vi "Plotmatrix Property Dialog.vi"(6 "Control Ref Queue":T9, 7 "Multimatrix Representation":T10, 8 "error in (no error)":errorcluster, 11 "2D Feather.lvclass in":refnum<class "XY Plot Matrix.lvclass">) -> (0 "error out":errorcluster, 3 "2D Feather.lvclass out":refnum<class "XY Plot Matrix.lvclass">, 4 "Cancel?":bool)   [LabVIEW 2020, in "XY Plot Matrix.lvclass"]
uses:
  <vilib>/Math Plots/2D Math Plots/XY Plot Matrix/XY Plot Matrix/XY Plot Matrix.lvclass
  e:/builds/penguin/labview/branches/2020/dev/dist/vi.lib/Math Plots/2D Math Plots/2D Plot/2D Plot/2D Plot.lvclass
  <vilib>/Math Plots/2D Math Plots/2D Plot/Action String/XYPlotMatrix Ctrl Act Queue.ctl
  <vilib>/Math Plots/2D Math Plots/2D Plot/Action String/XYPlotMatrix Ctrl Act Cluster.ctl
  <vilib>/Math Plots/2D Math Plots/2D Plot/Action String/2DMathPlot State Class.ctl
  <vilib>/Math Plots/2D Math Plots/2D Plot/2D Plot/Typedef/Scale Cluster.ctl
  <vilib>/Utility/miscctls.llb/LVOffsetAndMultiplierTypeDef.ctl
  <vilib>/Math Plots/2D Math Plots/XY Plot Matrix/XY Plot Matrix/Typedef/Plotmatrix Property Array.ctl
  <vilib>/Math Plots/2D Math Plots/XY Plot Matrix/XY Plot Matrix/Typedef/Plotmatrix Property.ctl
  <vilib>/Math Plots/2D Math Plots/2D Plot/2D Plot/Typedef/Plot Property Array.ctl
  <vilib>/Math Plots/2D Math Plots/2D Plot/2D Plot/Typedef/Plot Property.ctl
  <vilib>/Math Plots/2D Math Plots/2D Plot/2D Plot/Typedef/Graph General Property.ctl
  <vilib>/Math Plots/2D Math Plots/XY Plot Matrix/XY Plot Matrix/Typedef/Mulitmatrix Representation.ctl
  <vilib>/Math Plots/2D Math Plots/XY Plot Matrix/XY Plot Matrix/Typedef/Matrix Representation.ctl
  <vilib>/Math Plots/2D Math Plots/2D Plot/2D Plot/Typedef/Range Cluster.ctl
  <vilib>/Math Plots/2D Math Plots/2D Plot/2D Plot/Typedef/Temp Graph State.ctl
  <vilib>/Math Plots/2D Math Plots/2D Plot/2D Plot/Typedef/Temp Graph Data Action.ctl
  <vilib>/Math Plots/2D Math Plots/XY Plot Matrix/XY Plot Matrix/XY Plot Matrix.lvclass/XY Plot Matrix.ctl
  <vilib>/Math Plots/2D Math Plots/2D Plot/2D Plot/2D Plot.lvclass
panel:
  in  "Graph General":T1
  in  "Format String":string[](array[string])
  in  "Plotmatrix Property":T2
  in  "Scales Array":T6[](array[typedef])
  in  "Dialog Tab":enum32{"UI", "Input & Output"}(tab)
  in  "OK":bool
  in  "Cancel":bool
  in  "Help":bool
  in  "Page Tab":T8(tab)
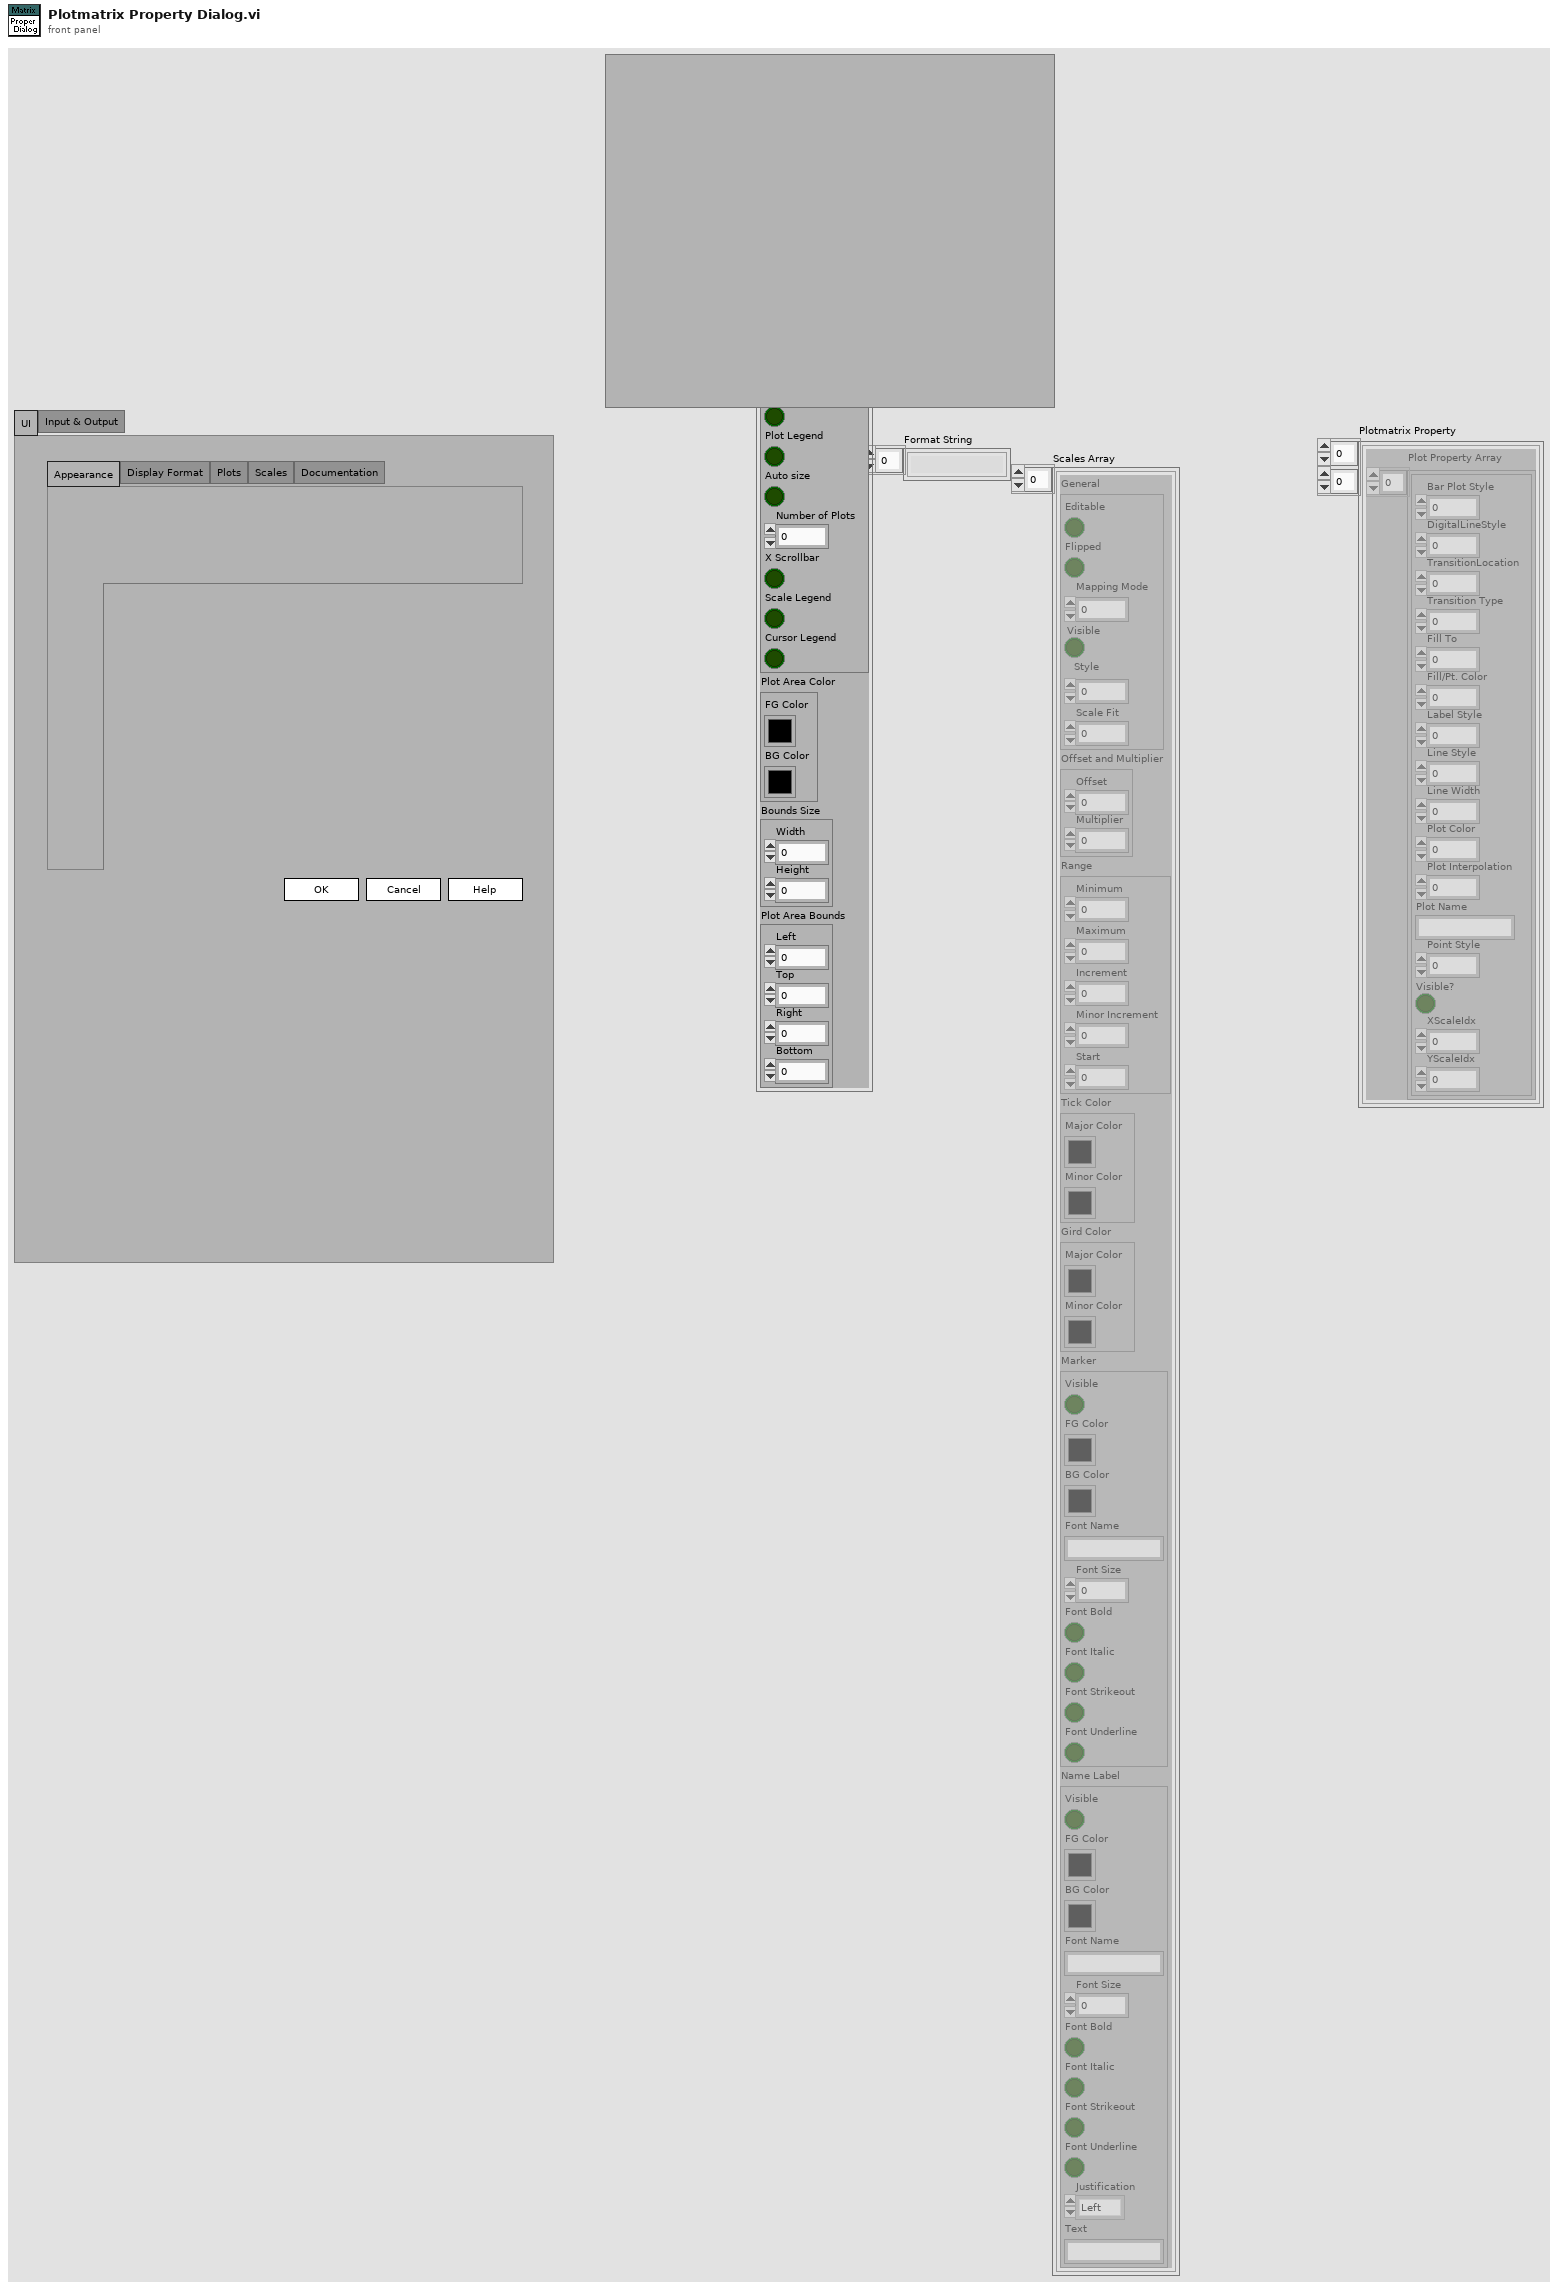
[diagram p1: front panel]
types:
  T1 = typedef "2D Plot.lvclass/Graph General Property.ctl" = cluster{"Palette Visible":cluster{"Graph Legend":bool, "Plot Legend":bool, "Auto size":bool, "Number of Plots":u32, "X Scrollbar":bool, "Scale Legend":bool, "Cursor Legend":bool}, "Plot Area Color":cluster{"FG Color":u32, "BG Color":u32}, "Bounds Size":cluster{"Width":u32, "Height":u32}, "Plot Area Bounds":cluster{"Left":i16, "Top":i16, "Right":i16, "Bottom":i16}}
  T2 = typedef "XY Plot Matrix.lvclass/Plotmatrix Property Array.ctl" = T3[][]
  T3 = typedef "XY Plot Matrix.lvclass/Plotmatrix Property.ctl" = cluster{"Plot Property Array":T4}
  T4 = typedef "2D Plot.lvclass/Plot Property Array.ctl" = T5[]
  T5 = typedef "2D Plot.lvclass/Plot Property.ctl" = cluster{"Bar Plot Style":u8, "DigitalLineStyle":u8, "TransitionLocation":u8, "Transition Type":u8, "Fill To":i16, "Fill/Pt. Color":u32, "Label Style":u8, "Line Style":u8, "Line Width":u8, "Plot Color":u32, "Plot Interpolation":u8, "Plot Name":string, "Point Style":u8, "Visible?":bool, "XScaleIdx":u32, "YScaleIdx":u32}
  T6 = typedef "2D Plot.lvclass/Scale Cluster.ctl" = cluster{"General":cluster{"Editable":bool, "Flipped":bool, "Mapping Mode":u8, "Visible":bool, "Style":u8, "Scale Fit":u8}, "Offset and Multiplier":T7, "Range":cluster{"Minimum":dbl, "Maximum":dbl, "Increment":dbl, "Minor Increment":dbl, "Start":dbl}, "Tick Color":cluster{"Major Color":u32, "Minor Color":u32}, "Gird Color":cluster{"Major Color":u32, "Minor Color":u32}, "Marker":cluster{"Visible":bool, "FG Color":u32, "BG Color":u32, "Font Name":string, "Font Size":u32, "Font Bold":bool, "Font Italic":bool, "Font Strikeout":bool, "Font Underline":bool}, "Name Label":cluster{"Visible":bool, "FG Color":u32, "BG Color":u32, "Font Name":string, "Font Size":u32, "Font Bold":bool, "Font Italic":bool, "Font Strikeout":bool, "Font Underline":bool, "Justification":enum16{"Left", "Center", "Right"}, "Text":string}}
  T7 = typedef "LVOffsetAndMultiplierTypeDef.ctl" = cluster{"Offset":dbl, "Multiplier":dbl}
  T8 = enum32{"Appearance", "Display Format", "Plots", "Scales", "Documentation"}
  T9 = typedef "XYPlotMatrix Ctrl Act Queue.ctl" = refnum<queue>
  T10 = typedef "XY Plot Matrix.lvclass/Mulitmatrix Representation.ctl" = cluster{"Matrix Representation Array":T11[][], "Max Range Array":T12[][], "Max Plot Number":i32}
  T11 = typedef "XY Plot Matrix.lvclass/Matrix Representation.ctl" = cluster{"Graph Matrix":cluster{"X":dbl[], "Y":dbl[]}[]}
  T12 = typedef "2D Plot.lvclass/Range Cluster.ctl" = cluster{"X Range":cluster{"Max X":dbl, "Min X":dbl}, "Y Range":cluster{"Max Y":dbl, "Min Y":dbl}}
  T13 = typedef "2D Plot.lvclass/Temp Graph State.ctl" = enum16{"Create", "Update Graph", "Update Property Only", "Get Plot Name", "Get Axis Name", "Destory"}
  T14 = typedef "2D Plot.lvclass/Temp Graph Data Action.ctl" = enum16{"Data Cluster", "Property Class", "Control Queue"}
  T15 = typedef "XYPlotMatrix Ctrl Act Cluster.ctl" = cluster{"Facade VI":refnum<vi>, "XControl":refnum<vi>, "Sub Panel":refnum<vi>, "Sub VI":refnum<vi>, "Export Image":refnum<vi>, "Display State Change Class":T16}
  T16 = typedef "2DMathPlot State Class.ctl" = enum16{"Update All (Undo)", "Update General", "Update Appearance", "Update Format", "Update Scale", "Update Marker", "Update Cursor", "None"}
  T17 = typedef "2D Plot.lvclass/Property Cluster.ctl" = cluster{"Graph General":T1, "Format Property":string[], "Scale Array":T18, "Cursor Property":T19, "Annotation List":T21, "Active Cursor":i32, "Active Plot":i32}
  T18 = typedef "2D Plot.lvclass/Scale Array.ctl" = T6[]
  T19 = typedef "2D Plot.lvclass/Cursor Property.ctl" = cluster{"Cursor List":T20, "Cursor List Addtional":cluster{"Cursor Selection Color":u32, "Line Style":u8, "Line Width":u8, "Visible":bool}[]}
  T20 = typedef "LVCursorListTypeDef.ctl" = cluster{"Name":string, "Color":u32, "Style":u8, "Point Style":u8, "Name Visible":bool, "Allow Drag":bool, "Cursor Mode":u32, "Plot":i32, "Index":i32, "Position":cluster{"X":dbl, "Y":dbl}, "X Scale":u32, "Y Scale":u32, "Watch Plots":i32[], "Watch All Plots":bool, "Plot Area":i32, "Label Offset":cluster{"X":dbl, "Y":dbl}}[]
  T21 = typedef "LVAnnotationListTypeDef.ctl" = cluster{"Name":string, "Color":u32, "Style":u8, "Point Style":u8, "Name Visible":bool, "Allow Drag":bool, "Annotation Mode":u32, "Plot":i32, "Index":i32, "Position":cluster{"X":dbl, "Y":dbl}, "X Scale":u32, "Y Scale":u32, "Show Arrow":bool, "Lock Name":bool, "Plot Area":i32, "Label Offset":cluster{"X":dbl, "Y":dbl}}[]
  T22 = enum8{"Enabled", "Disabled", "Disabled and Grayed Out"}
  T23 = enum32{"Bad", "Idle", "Run top level", "Running"}[]
  T24 = enum32{"Bad", "Idle", "Run top level", "Running"}
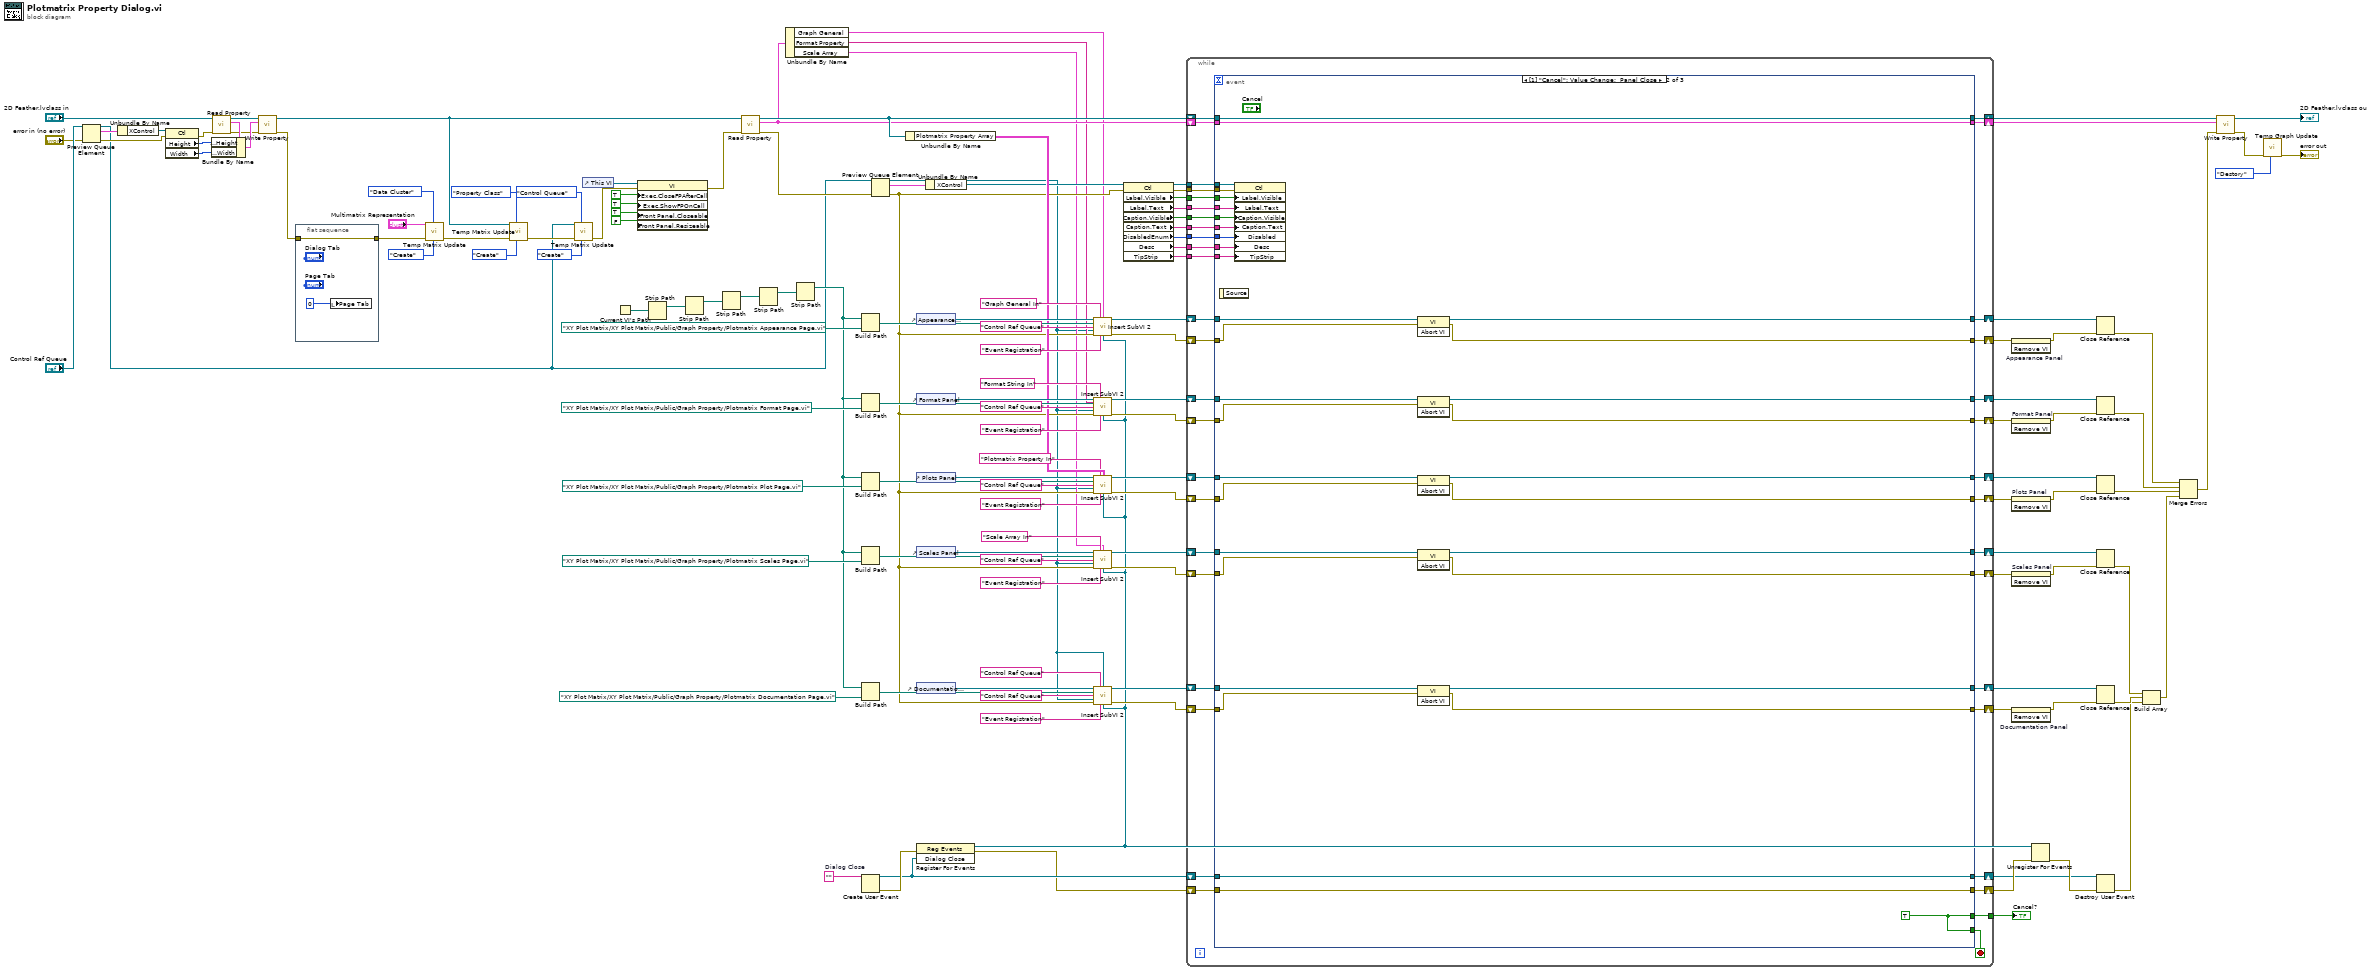
[diagram p0: block diagram]
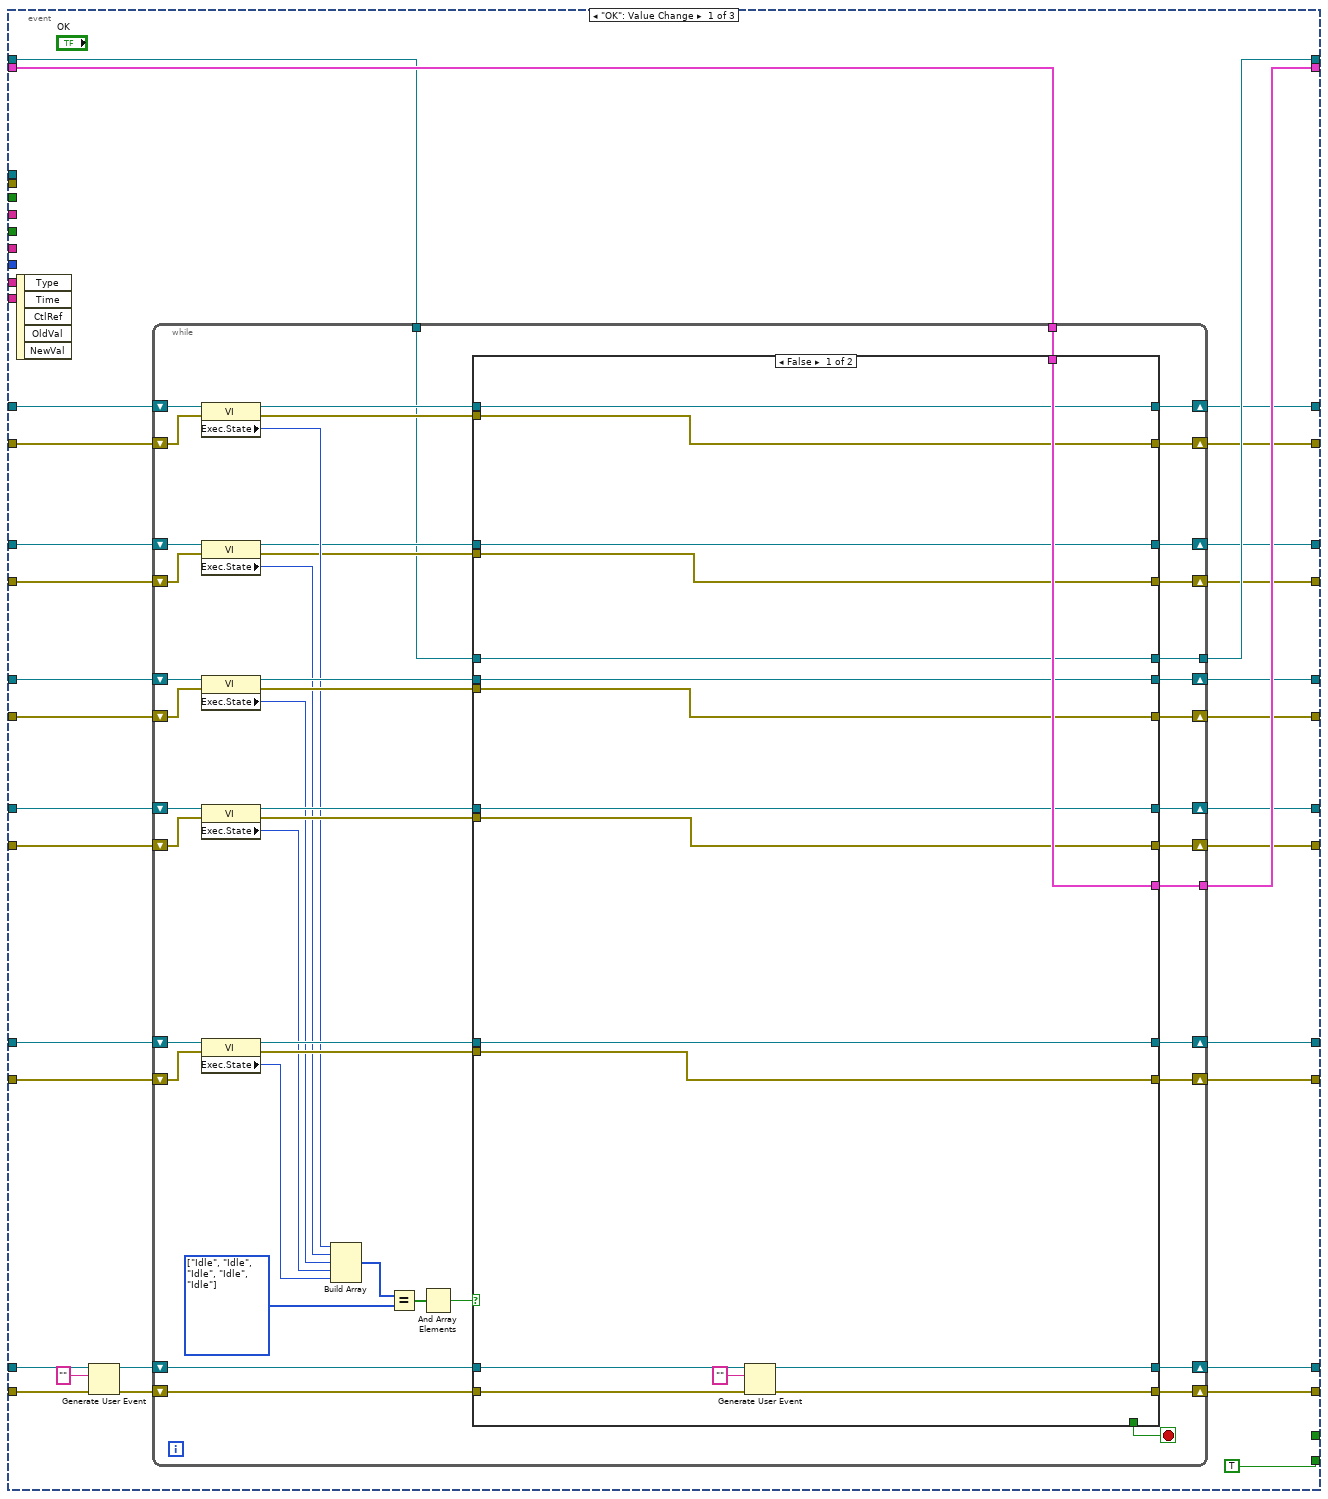
[diagram p2: hidden frame]
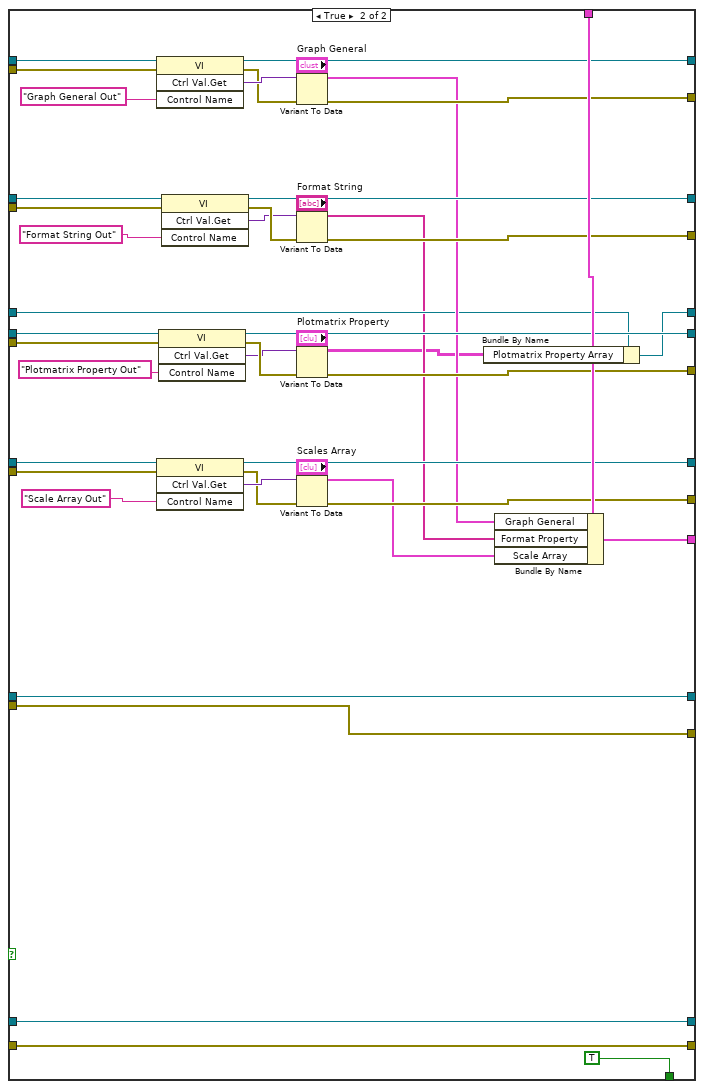
[diagram p3: hidden frame]
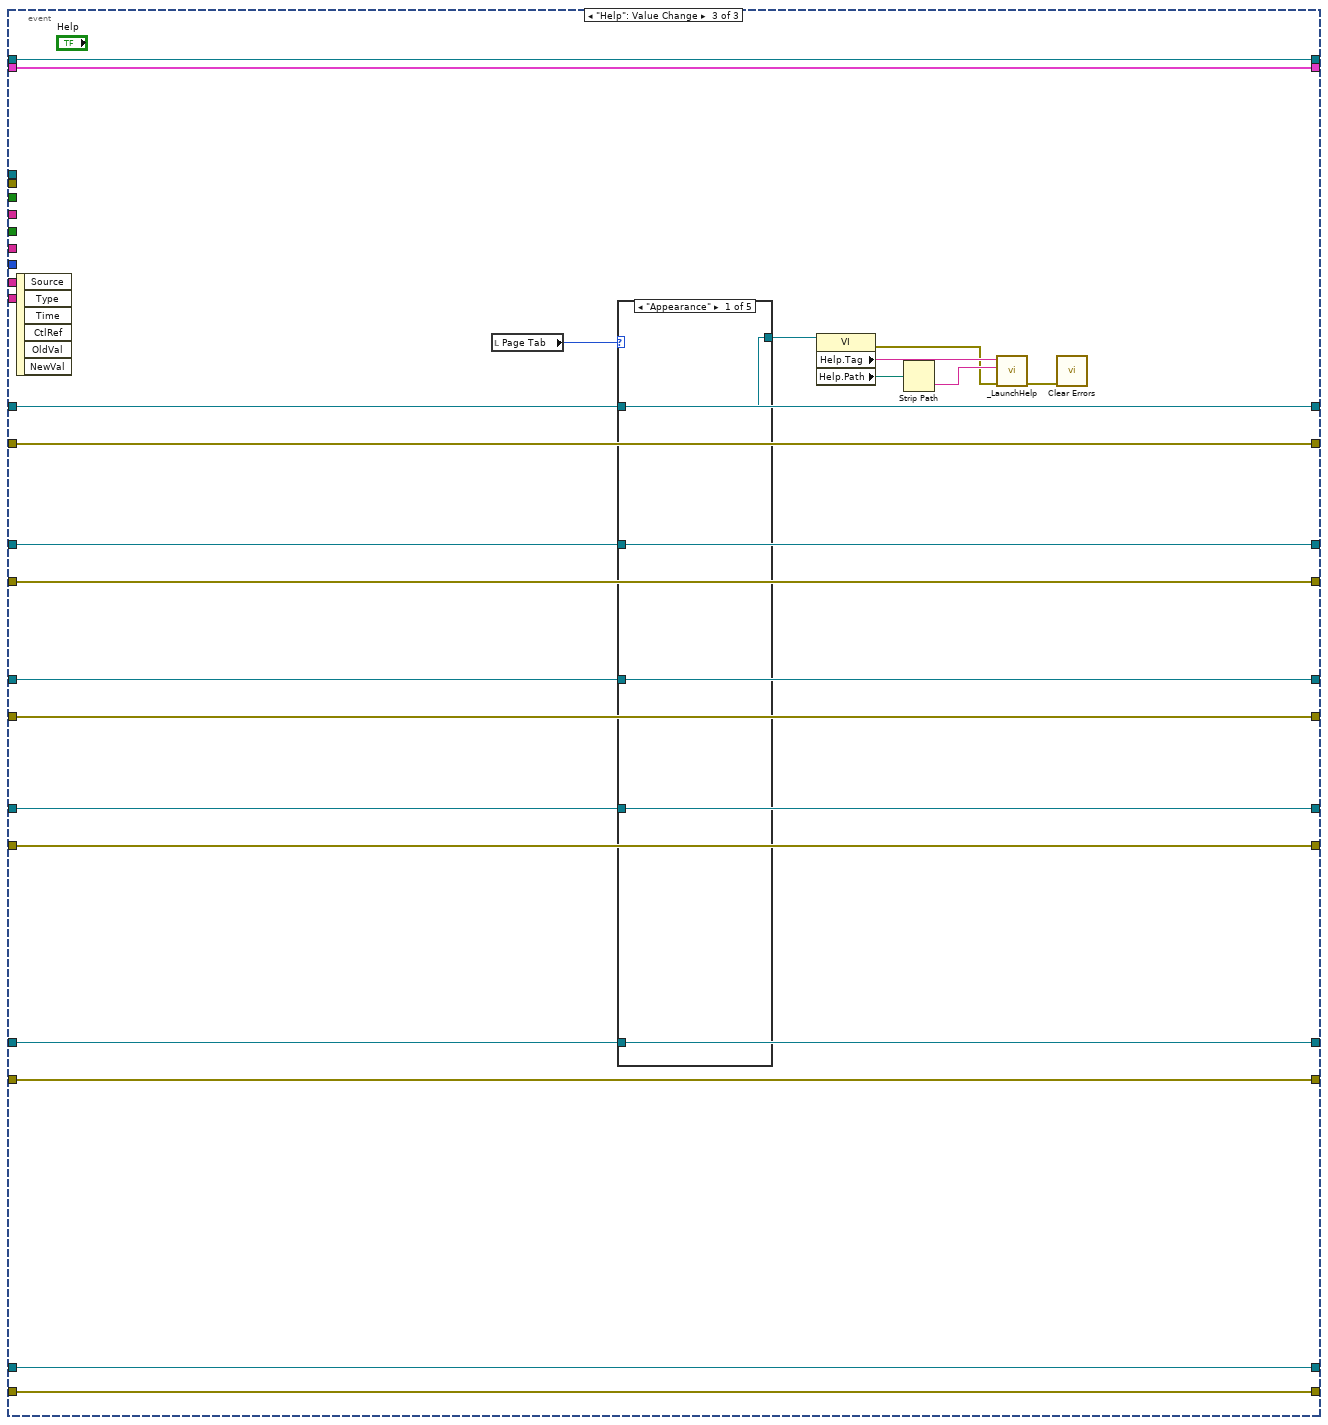
[diagram p4: hidden frame]
diagram:
  w121 = ""  # Dialog Close
  n1 = Preview Queue Element(queue="Control Ref Queue", error in (no error)="error in (no error)") -> (queue out=w14:T9, element=w24:T15, error out=w16:errorcluster)  [unwired: 2 out]
  n2 = Unbundle By Name(w24) -> ("XControl"=w23:refnum<vi>)
  n3 = property class="Ctl"(reference=w23, error in=w16) -> (error out=w13:errorcluster, "Height"=w9:u32, "Width"=w8:u32)  [unwired: 1 out]
  n4 = call <vilib>:"Read Property.vi"("error in (no error)"=w13, "2D Plot.lvclass in"="2D Feather.lvclass in") -> ("error out"=w12:errorcluster, "XY Graph Property Cluster"=w20:T17, "2D Plot.lvclass out"=w21:refnum<class "XY Plot Matrix.lvclass">)  [unwired: 7 out]
  n5 = Bundle By Name(cluster=w20, "Graph General.Bounds Size.Height"=w9, "Graph General.Bounds Size.Width"=w8) -> (w19:T17)
  n6 = call <vilib>:"Write Property.vi"("error in (no error)"=w12, "XY Graph Property Cluster"=w19, "2D Plot.lvclass in"=w21) -> ("error out"=w10:errorcluster, "2D Plot.lvclass out"=w17:refnum<class "XY Plot Matrix.lvclass">)  [unwired: 7 out]
  n7 = flat-sequence {
    tunnel: w10 -> [w138]
    tunnel: [w138] -> w3
    frame #0 {
      n8 = local write "Page Tab"(u32 0) -> ()
    }
  }
  n9 = call <vilib>:"Temp Matrix Update.vi"("State"=Temp_Graph_State."Create", "Data Name"=Temp_Graph_Data_Action."Data Cluster", "error in (no error)"=w3, "Property In"="Multimatrix Representation") -> ("error out"=w2:errorcluster)  [unwired: 1 in, 6 out]
  n10 = call <vilib>:"Temp Matrix Update.vi"("State"=Temp_Graph_State."Create", "Data Name"=Temp_Graph_Data_Action."Property Class", "error in (no error)"=w2, "Property In"=w17) -> ("error out"=w39:errorcluster)  [unwired: 1 in, 6 out]
  n11 = call <vilib>:"Temp Matrix Update.vi"("State"=Temp_Graph_State."Create", "Data Name"=Temp_Graph_Data_Action."Control Queue", "error in (no error)"=w39, "Property In"=w14) -> ("error out"=w36:errorcluster)  [unwired: 1 in, 6 out]
  n12 = control-ref of="This VI"() -> (w137:refnum<vi>)
  n13 = Current VI's Path() -> (path=w129:path)
  n14 = property class="VI"(reference=w137, error in=w36, "Exec.CloseFPAfterCall"=TRUE ("Execution:Close After Call"), "Exec.ShowFPOnCall"=TRUE ("Execution:Show Front Panel On Call"), "Front Panel.Closeable"=TRUE ("Front Panel Window:Closeable"), "Front Panel.Resizeable"=FALSE ("Front Panel Window:Resizeable")) -> (error out=w127:errorcluster)  [unwired: 1 out]
  n15 = Strip Path(path=w129) -> (stripped path=w130:path)  [unwired: 1 out]
  n16 = Strip Path(path=w130) -> (stripped path=w131:path)  [unwired: 1 out]
  n17 = Strip Path(path=w131) -> (stripped path=w128:path)  [unwired: 1 out]
  n18 = call <vilib>:"Read Property.vi"("error in (no error)"=w127, "2D Plot.lvclass in"=w17) -> ("error out"=w51:errorcluster, "XY Graph Property Cluster"=w93:T17, "2D Plot.lvclass out"=w94:refnum<class "XY Plot Matrix.lvclass">)  [unwired: 7 out]
  n19 = Strip Path(path=w128) -> (stripped path=w27:path)  [unwired: 1 out]
  n20 = Unbundle By Name(w93) -> ("Graph General"=w22:T1, "Format Property"=w29:string[], "Scale Array"=w28:T18)
  n21 = Strip Path(path=w27) -> (stripped path=w26:path)  [unwired: 1 out]
  n22 = Build Path(base path=w26, name or relative path=path "XY Plot Matrix/XY Plot Matrix/Public/Graph Property/Plotmatrix Appearance Page.vi") -> (appended path=w126:path)
  n23 = Build Path(base path=w26, name or relative path=path "XY Plot Matrix/XY Plot Matrix/Public/Graph Property/Plotmatrix Format Page.vi") -> (appended path=w117:path)
  n24 = Build Path(base path=w26, name or relative path=path "XY Plot Matrix/XY Plot Matrix/Public/Graph Property/Plotmatrix Plot Page.vi") -> (appended path=w97:path)
  n25 = Build Path(base path=w26, name or relative path=path "XY Plot Matrix/XY Plot Matrix/Public/Graph Property/Plotmatrix Scales Page.vi") -> (appended path=w111:path)
  n26 = Build Path(base path=w26, name or relative path=path "XY Plot Matrix/XY Plot Matrix/Public/Graph Property/Plotmatrix Documentation Page.vi") -> (appended path=w99:path)
  n27 = Create User Event(user event datatype=w121) -> (user event=w82:refnum<user-event>, error out=w122:errorcluster)  [unwired: 1 in]
  n28 = Preview Queue Element(queue=w14, error in (no error)=w51) -> (queue out=w25:T9, element=w50:T15, error out=w32:errorcluster)  [unwired: 2 out]
  n29 = Unbundle By Name(w94) -> ("Plotmatrix Property Array"=w101:T2)
  n30 = control-ref of="Appearance Panel"() -> (w125:refnum<vi>)
  n31 = control-ref of="Format Panel"() -> (w118:refnum<vi>)
  n32 = control-ref of="Plots Panel"() -> (w104:refnum<vi>)
  n33 = control-ref of="Scales Panel"() -> (w113:refnum<vi>)
  n34 = control-ref of="Documentation Panel"() -> (w107:refnum<vi>)
  n35 = register-events(error in=w122, w82) -> (reference out=w31:refnum<event-registration>, error out=w81:errorcluster)  [unwired: 1 in]
  n36 = Unbundle By Name(w50) -> ("XControl"=w49:refnum<vi>)
  n37 = call <vilib>:"Insert SubVI 2.vi"("Sub Panel Ref"=w125, "Label 1"="Graph General In", "Value 1"=w22, "VI Path"=w126, "Label 3"="Control Ref Queue" ("Label 1"), "Value 3"=w25, "error in (no error)"=w32, "Label 2"="Event Registration", "Value 2"=w31) -> ("vi reference"=w92:refnum<vi>, "error out"=w87:errorcluster)  [unwired: 5 out]
  n38 = call <vilib>:"Insert SubVI 2.vi"("Sub Panel Ref"=w118, "Label 1"="Format String In" ("Label 2"), "Value 1"=w29, "VI Path"=w117, "Label 3"="Control Ref Queue" ("Label 1"), "Value 3"=w25, "error in (no error)"=w32, "Label 2"="Event Registration", "Value 2"=w31) -> ("vi reference"=w91:refnum<vi>, "error out"=w86:errorcluster)  [unwired: 5 out]
  n39 = call <vilib>:"Insert SubVI 2.vi"("Sub Panel Ref"=w104, "Label 1"="Plotmatrix Property In", "Value 1"=w101, "VI Path"=w97, "Label 3"="Control Ref Queue" ("Label 1"), "Value 3"=w25, "error in (no error)"=w32, "Label 2"="Event Registration", "Value 2"=w31) -> ("vi reference"=w90:refnum<vi>, "error out"=w85:errorcluster)  [unwired: 5 out]
  n40 = call <vilib>:"Insert SubVI 2.vi"("Sub Panel Ref"=w113, "Label 1"="Scale Array In", "Value 1"=w28, "VI Path"=w111, "Label 3"="Control Ref Queue" ("Label 1"), "Value 3"=w25, "error in (no error)"=w32, "Label 2"="Event Registration", "Value 2"=w31) -> ("vi reference"=w89:refnum<vi>, "error out"=w84:errorcluster)  [unwired: 5 out]
  n41 = call <vilib>:"Insert SubVI 2.vi"("Sub Panel Ref"=w107, "Label 1"="Control Ref Queue", "Value 1"=w25, "VI Path"=w99, "Label 3"="Control Ref Queue" ("Label 1"), "Value 3"=w25, "error in (no error)"=w32, "Label 2"="Event Registration", "Value 2"=w31) -> ("vi reference"=w88:refnum<vi>, "error out"=w83:errorcluster)  [unwired: 5 out]
  n42 = property class="Ctl"(reference=w49, error in=w32) -> (reference out=w48:refnum<vi>, error out=w47:errorcluster, "Label.Visible"=w46:bool, "Label.Text"=w45:string, "Caption.Visible"=w44:bool, "Caption.Text"=w43:string, "DisabledEnum"=w42:T22, "Desc"=w41:string, "TipStrip"=w40:string)
  n43 = while {
    shift-right: [w164] -> w78
    shift-left: w94 -> [w178]
    shift-right: [w163] -> w79
    shift-left: w93 -> [w177]
    shift-right: [w162] -> w70
    shift-left: w87 -> [w171]
    shift-right: [w161] -> w68
    shift-left: w86 -> [w170]
    shift-right: [w160] -> w62
    shift-left: w85 -> [w169]
    shift-right: [w159] -> w59
    shift-left: w84 -> [w168]
    shift-right: [w158] -> w57
    shift-left: w83 -> [w167]
    shift-right: [w157] -> w54
    shift-left: w81 -> [w165]
    shift-right: [w151] -> w52
    shift-left: w82 -> [w166]
    shift-right: [w152] -> w56
    shift-left: w88 -> [w172]
    shift-right: [w153] -> w61
    shift-left: w89 -> [w173]
    shift-right: [w154] -> w63
    shift-left: w90 -> [w174]
    shift-right: [w155] -> w66
    shift-left: w91 -> [w175]
    shift-right: [w156] -> w71
    shift-left: w92 -> [w176]
    tunnel: [w149] -> w80
    tunnel: w48 -> [w148]
    tunnel: w47 -> [w147]
    tunnel: w46 -> [w146]
    tunnel: w45 -> [w145]
    tunnel: w44 -> [w144]
    tunnel: w43 -> [w143]
    tunnel: w42 -> [w142]
    tunnel: w41 -> [w141]
    tunnel: w40 -> [w140]
    stop <- w150 stop-if-true
    n44 = event shown="[1] \"Cancel\": Value Change;  Panel Close" {
      selector: _ -> [_ _ _]
      dyn-events: _ -> [_ _ _]
      timeout: _ -> [_ _ _]
      tunnel: w178 -> [w194 w331 w367]
      tunnel: w177 -> [w195 w332 w368]
      tunnel: w176 -> [w210 w354 w359]
      tunnel: w175 -> [w209 w350 w358]
      tunnel: w174 -> [w208 w348 w357]
      tunnel: w173 -> [w207 w346 w356]
      tunnel: w172 -> [w206 w344 w355]
      tunnel: w171 -> [w205 w353 w375]
      tunnel: w170 -> [w204 w349 w374]
      tunnel: w169 -> [w203 w347 w373]
      tunnel: w168 -> [w202 w345 w372]
      tunnel: w167 -> [w201 w343 w371]
      tunnel: w166 -> [w197 w334 w369]
      tunnel: w165 -> [w198 w333 w370]
      tunnel: [w193 w331 w367] -> w164
      tunnel: [w192 w332 w368] -> w163
      tunnel: [w191 w351 w375] -> w162
      tunnel: [w190 w341 w374] -> w161
      tunnel: [w179 w339 w373] -> w160
      tunnel: [w180 w337 w372] -> w159
      tunnel: [w189 w335 w371] -> w158
      tunnel: [w188 w333 w370] -> w157
      tunnel: [w187 w352 w359] -> w156
      tunnel: [w186 w342 w358] -> w155
      tunnel: [w185 w340 w357] -> w154
      tunnel: [w184 w338 w356] -> w153
      tunnel: [w183 w336 w355] -> w152
      tunnel: [w181 w334 w369] -> w151
      tunnel: [TRUE w321 _] -> w150
      tunnel: [_ w321 _] -> w149
      tunnel: w148 -> [_ w330 _]
      tunnel: w147 -> [_ w329 _]
      tunnel: w146 -> [_ w328 _]
      tunnel: w145 -> [_ w327 _]
      tunnel: w144 -> [_ w326 _]
      tunnel: w143 -> [_ w325 _]
      tunnel: w142 -> [_ w324 _]
      tunnel: w141 -> [_ w323 _]
      tunnel: w140 -> [_ w322 _]
      event "OK": Value Change {
        n45 = event-data() -> ()  [unwired: 6 out]
        n46 = Generate User Event(user event=w197, event data cluster="" ("event data"), error in=w198) -> (user event out=w196:refnum<user-event>, error out=w199:errorcluster)  [unwired: 1 in]
        n47 = while {
          tunnel: w195 -> [w258]
          tunnel: [w257] -> w192
          shift-right: [w224] -> w181
          shift-left: w196 -> [w225]
          shift-right: [w215] -> w188
          shift-left: w199 -> [w217]
          tunnel: w194 -> [w214]
          tunnel: [w213] -> w193
          shift-right: [w235] -> w189
          shift-left: w201 -> [w231]
          shift-right: [w234] -> w183
          shift-left: w206 -> [w230]
          shift-right: [w212] -> w180
          shift-left: w202 -> [w239]
          shift-right: [w236] -> w184
          shift-left: w207 -> [w240]
          shift-right: [w242] -> w185
          shift-left: w208 -> [w245]
          shift-right: [w211] -> w179
          shift-left: w203 -> [w241]
          shift-right: [w219] -> w186
          shift-left: w209 -> [w222]
          shift-right: [w218] -> w190
          shift-left: w204 -> [w223]
          shift-right: [w256] -> w187
          shift-left: w210 -> [w254]
          shift-right: [w255] -> w191
          shift-left: w205 -> [w252]
          stop <- w246 stop-if-true
          w249 = T23 [enum."Idle", enum."Idle", enum."Idle", enum."Idle", enum."Idle"] items=["Bad", "Idle", "Run top level", "Running"]
          n48 = property class="VI"(reference=w254, error in=w252) -> (reference out=w253:refnum<vi>, error out=w251:errorcluster, "Exec.State"=w229:T24)
          n49 = property class="VI"(reference=w222, error in=w223) -> (reference out=w221:refnum<vi>, error out=w220:errorcluster, "Exec.State"=w216:T24)
          n50 = property class="VI"(reference=w245, error in=w241) -> (reference out=w244:refnum<vi>, error out=w243:errorcluster, "Exec.State"=w228:T24)
          n51 = property class="VI"(reference=w240, error in=w239) -> (reference out=w238:refnum<vi>, error out=w237:errorcluster, "Exec.State"=w227:T24)
          n52 = property class="VI"(reference=w230, error in=w231) -> (reference out=w232:refnum<vi>, error out=w233:errorcluster, "Exec.State"=w226:T24)
          n53 = Build Array(w229, w216, w228, w227, w226) -> (w250:T23)
          n54 = Equal?(x=w250, y=w249) -> (x = y?=w248:bool[])
          n55 = And Array Elements(Boolean array=w248) -> (logical AND=w247:bool)
          n56 = case shown="False" w247 {
            tunnel: w258 -> [w275 w320]
            tunnel: [w275 w319] -> w257
            tunnel: [w274 w315] -> w256
            tunnel: [w273 w314] -> w255
            tunnel: w253 -> [w274 w313]
            tunnel: w251 -> [w273 w312]
            tunnel: [_ TRUE] -> w246
            tunnel: w244 -> [w271 w306]
            tunnel: w243 -> [w272 w307]
            tunnel: [w272 w305] -> w211
            tunnel: [w271 w304] -> w242
            tunnel: w238 -> [w269 w300]
            tunnel: w237 -> [w270 w299]
            tunnel: [w269 w298] -> w236
            tunnel: [w270 w297] -> w212
            tunnel: w232 -> [w268 w280]
            tunnel: w233 -> [w267 w279]
            tunnel: [w268 w280] -> w234
            tunnel: [w267 w279] -> w235
            tunnel: w225 -> [w266 w296]
            tunnel: [w265 w296] -> w224
            tunnel: w221 -> [w263 w292]
            tunnel: w220 -> [w262 w291]
            tunnel: [w263 w290] -> w219
            tunnel: [w262 w289] -> w218
            tunnel: w217 -> [w261 w288]
            tunnel: [w260 w288] -> w215
            tunnel: w214 -> [w259 w284]
            tunnel: [w259 w281] -> w213
            frame False {
              n57 = Generate User Event(user event=w266, event data cluster="" ("event data"), error in=w261) -> (user event out=w265:refnum<user-event>, error out=w260:errorcluster)  [unwired: 1 in]
            }
            frame True {
              n58 = invoke class="VI" method="Ctrl Val.Get"(reference=w313, error in=w312, "Control Name"="Graph General Out") -> (reference out=w315:refnum<vi>, error out=w316:errorcluster, "Get Control Value Variant"=w317:variant)  [unwired: 1 in, 1 out]
              n59 = invoke class="VI" method="Ctrl Val.Get"(reference=w300, error in=w299, "Control Name"="Scale Array Out") -> (reference out=w298:refnum<vi>, error out=w301:errorcluster, "Get Control Value Variant"=w302:variant)  [unwired: 1 in, 1 out]
              n60 = invoke class="VI" method="Ctrl Val.Get"(reference=w306, error in=w307, "Control Name"="Plotmatrix Property Out") -> (reference out=w304:refnum<vi>, error out=w310:errorcluster, "Get Control Value Variant"=w309:variant)  [unwired: 1 in, 1 out]
              n61 = invoke class="VI" method="Ctrl Val.Get"(reference=w292, error in=w291, "Control Name"="Format String Out") -> (reference out=w290:refnum<vi>, error out=w295:errorcluster, "Get Control Value Variant"=w294:variant)  [unwired: 1 in, 1 out]
              n62 = Variant To Data(error in=w316, type="Graph General", Variant=w317) -> (data=w286:T1, error out=w314:errorcluster)
              n63 = Variant To Data(error in=w295, type="Format String", Variant=w294) -> (data=w277:string[], error out=w289:errorcluster)
              n64 = Variant To Data(error in=w310, type="Plotmatrix Property", Variant=w309) -> (data=w276:T2, error out=w305:errorcluster)
              n65 = Variant To Data(error in=w301, type="Scales Array", Variant=w302) -> (data=w278:T6[], error out=w297:errorcluster)
              n66 = Bundle By Name(cluster=w284, "Plotmatrix Property Array"=w276) -> (w281:refnum<class "XY Plot Matrix.lvclass">)
              n67 = Bundle By Name(cluster=w320, "Graph General"=w286, "Format Property"=w277, "Scale Array"=w278) -> (w319:T17)
            }
          }
        }
      }
      event "Cancel": Value Change; Panel Close {
        w321 = TRUE
        n68 = event-data() -> ()  [unwired: 2 out]
        n69 = property class="Ctl"(reference=w330, error in=w329, "Label.Visible"=w328, "Label.Text"=w327, "Caption.Visible"=w326, "Caption.Text"=w325, "Disabled"=w324, "Desc"=w323, "TipStrip"=w322) -> ()  [unwired: 2 out]
        n70 = invoke class="VI" method="Abort VI"(reference=w354, error in=w353) -> (reference out=w352:refnum<vi>, error out=w351:errorcluster)  [unwired: 1 in, 1 out]
        n71 = invoke class="VI" method="Abort VI"(reference=w350, error in=w349) -> (reference out=w342:refnum<vi>, error out=w341:errorcluster)  [unwired: 1 in, 1 out]
        n72 = invoke class="VI" method="Abort VI"(reference=w348, error in=w347) -> (reference out=w340:refnum<vi>, error out=w339:errorcluster)  [unwired: 1 in, 1 out]
        n73 = invoke class="VI" method="Abort VI"(reference=w346, error in=w345) -> (reference out=w338:refnum<vi>, error out=w337:errorcluster)  [unwired: 1 in, 1 out]
        n74 = invoke class="VI" method="Abort VI"(reference=w344, error in=w343) -> (reference out=w336:refnum<vi>, error out=w335:errorcluster)  [unwired: 1 in, 1 out]
      }
      event "Help": Value Change {
        n75 = event-data() -> ()  [unwired: 7 out]
        n76 = local read "Page Tab"() -> (w360:T8)
        n77 = case shown="\"Appearance\"" w360 {
          tunnel: w359 -> [w376 _ _ _ _]
          tunnel: [w376 w377 w378 w379 w380] -> w361
          tunnel: w358 -> [_ w377 _ _ _]
          tunnel: w357 -> [_ _ w378 _ _]
          tunnel: w356 -> [_ _ _ w379 _]
          tunnel: w355 -> [_ _ _ _ w380]
          frame "Appearance" {
          }
          frame "Display Format" {
          }
          frame "Plots" {
          }
          frame "Scales" {
          }
          frame "Documentation" {
          }
        }
        n78 = property class="VI"(reference=w361) -> (error out=w363:errorcluster, "Help.Tag"=w365:string, "Help.Path"=w366:path)  [unwired: 1 in, 1 out]
        n79 = Strip Path(path=w366) -> (name=w364:string)  [unwired: 1 out]
        n80 = call <helpdir>:"_LaunchHelp.vi"("error in (no error)"=w363, "CHM or HLP filename (lvdialog.chm)"=w364, "HTML filename"=w365) -> ("error out"=w362:errorcluster)  [unwired: 4 out]
        n81 = call <vilib>:"Clear Errors.vi"("error in (no error)"=w362) -> ()  [unwired: 5 in, 2 out]
      }
    }
  }
  "Cancel?" <- w80
  n82 = invoke on="Appearance Panel" class="SubPnl" method="Remove VI"(error in=w70) -> (error out=w69:errorcluster)  [unwired: 2 in, 2 out]
  n83 = invoke on="Format Panel" class="SubPnl" method="Remove VI"(error in=w68) -> (error out=w67:errorcluster)  [unwired: 2 in, 2 out]
  n84 = invoke on="Plots Panel" class="SubPnl" method="Remove VI"(error in=w62) -> (error out=w64:errorcluster)  [unwired: 2 in, 2 out]
  n85 = invoke on="Scales Panel" class="SubPnl" method="Remove VI"(error in=w59) -> (error out=w60:errorcluster)  [unwired: 2 in, 2 out]
  n86 = invoke on="Documentation Panel" class="SubPnl" method="Remove VI"(error in=w57) -> (error out=w58:errorcluster)  [unwired: 2 in, 2 out]
  n87 = Unregister For Events(event registration refnum=w31, error in=w54) -> (error out=w53:errorcluster)
  n88 = Close Reference(reference=w71, error in (no error)=w69) -> (error out=w65:errorcluster)
  n89 = Close Reference(reference=w66, error in (no error)=w67) -> (error out=w75:errorcluster)
  n90 = Close Reference(reference=w63, error in (no error)=w64) -> (error out=w74:errorcluster)
  n91 = Close Reference(reference=w61, error in (no error)=w60) -> (error out=w76:errorcluster)
  n92 = Close Reference(reference=w56, error in (no error)=w58) -> (error out=w72:errorcluster)
  n93 = Destroy User Event(user event=w52, error in=w53) -> (error out=w30:errorcluster)
  n94 = Build Array(w76, w72, w30) -> (w73:errorcluster[])
  n95 = Merge Errors(w65, w75, w74, w73) -> (w55:errorcluster)
  n96 = call <vilib>:"Write Property.vi"("error in (no error)"=w55, "XY Graph Property Cluster"=w79, "2D Plot.lvclass in"=w78) -> ("error out"=w35:errorcluster, "2D Plot.lvclass out"=→"2D Feather.lvclass out":refnum<class "XY Plot Matrix.lvclass">)  [unwired: 7 out]
  n97 = call <vilib>:"Temp Graph Update.vi"("State"=Temp_Graph_State."Destory", "error in (no error)"=w35) -> ("error out"=→"error out":errorcluster)  [unwired: 3 in, 6 out]
